vi "7_1.vi"   [LabVIEW 2020]
types:
  T1 = enum16{"open", "replace", "create", "open or create", "replace or create", "replace or create with confirmation"}
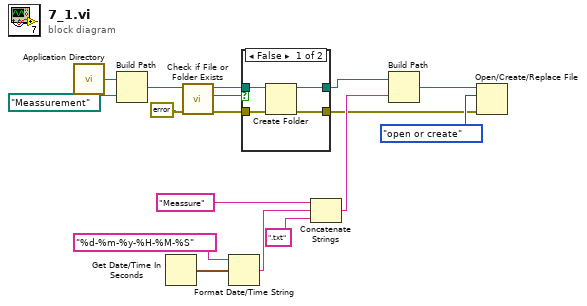
[diagram p0: block diagram]
diagram:
  n1 = call <vilib>:"Application Directory.vi"() -> ("Application Directory"=w16:path)
  n2 = Build Path(base path=w16, name or relative path=path "Meassurement" ("Name oder relativer Pfad")) -> (appended path=w13:path)
  n3 = Get Date/Time In Seconds() -> (seconds since 1Jan1904=w11:timestamp)
  n4 = call <vilib>:"Check if File or Folder Exists.vi"("error in (no error)"=errorcluster {"status"=FALSE, "code"=0, "source"=""}, "path"=w13) -> ("error out"=w3:errorcluster, "file or folder exists?"=w14:bool)  [unwired: 7 in, 1 out]
  n5 = Format Date/Time String(time format string (%c)="%d-%m-%y-%H-%M-%S" ("Zeitformatierungs-String (%c)"), seconds (now)=w11) -> (date/time string=w10:string)  [unwired: 1 in]
  n6 = case shown="False" w14 {
    tunnel: w13 -> [w20 w22]
    tunnel: [w19 w22] -> w1
    tunnel: [w18 w21] -> w4
    tunnel: w3 -> [w17 w21]
    frame False {
      n7 = Create Folder(path (use dialog)=w20, error in=w17) -> (created path=w19:path, error out=w18:errorcluster)  [unwired: 1 in, 1 out]
    }
    frame True {
    }
  }
  n8 = Concatenate Strings("Meassure", w10, ".txt" ("String")) -> (w8:string)
  n9 = Build Path(base path=w1, name or relative path=w8) -> (appended path=w6:path)
  n10 = Open/Create/Replace File(file path (use dialog)=w6, error in=w4, operation (0:open)=T1."open or create" ("Operation (0:open)")) -> ()  [unwired: 3 in, 3 out]
